vi "DataAndTime.vi"() -> ()   [LabVIEW 2020]
panel:
  in  "stop":bool
  in  "time stamp":timestamp
  in  "time format string (%c)":string
  out "date/time string":string
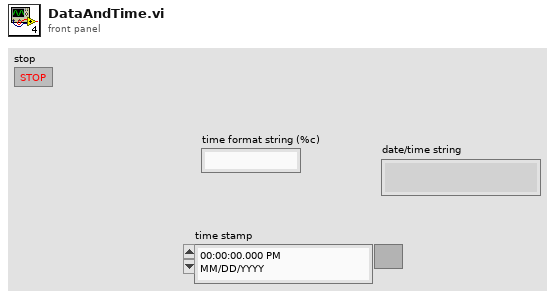
[diagram p1: front panel]
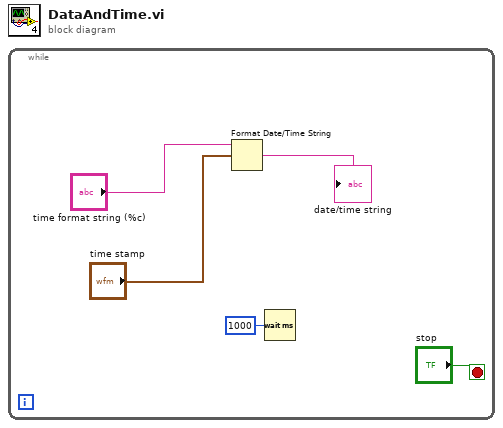
[diagram p0: block diagram]
diagram:
  n1 = while {
    stop <- "stop" stop-if-true
    n2 = Format Date/Time String(time format string (%c)="time format string (%c)", seconds (now)="time stamp") -> (date/time string=→"date/time string":string)  [unwired: 1 in]
    n3 = Wait (ms)(milliseconds to wait=u32 1000) -> ()  [unwired: 1 out]
  }
